vi "CS-4 Recall.vi"(8 "error in (no error)":errorcluster, 11 "VISA session":refnum<visa-resource-name>) -> (0 "error out":errorcluster, 1 "sweep rates":T2={"rate 0"=0.5, "rate 1"=0.25, "rate 2"=0.125, "rate 3"=10.0} {"rate 3" min=0.0 max=100.0 step=1.0 format="%.4f"; "rate 2" min=0.0 max=100.0 step=0.05 format="%.4f"; "rate 1" min=0.0 max=100.0 step=0.05 format="%.4f"; "rate 0" min=0.0 max=100.0 step=0.05 format="%.4f"}, 2 "range":cluster{"range 0":dbl, "range 1":dbl}={"range 0"=60.0, "range 1"=85.0} {"range 1" min=0.0 max=1000.0 format="%.3f"; "range 0" min=0.0 max=1000.0 step=1.0 format="%.3f"}, 3 "dup VISA session":refnum<visa-resource-name>, 4 "limits":T1={"Lower Current Limit"=-10.0, "Upper Current Limit"=10.0, "Voltage Limit"=5.0} {"Voltage Limit" min=0.0 max=5.0 format="%.2f"; "Upper Current Limit" min=-1000.0 max=1000.0 format="%.2f"; "Lower Current Limit" min=-1000.0 max=1000.0 format="%.1f"}, 5 "Units":enum16{"Amps", "Kilogauss", "Tesla"}(ring))   [LabVIEW 2016]
doc: "CS-4 Recall.vi uses the CS-4 driver VI's to recall setup information from a CS-4. This information includes display units, current sweep limits, and voltage limits. \n\nA VISA channel must be opened using CS-4 Initialize.vi before this VI is invoked."
panel:
  out "max supply current":dbl=100.0 format="%.3f"
  out "range 2 start":dbl format="%.3f"
  out "range 1 start":dbl format="%.3f"
  out "Cryo Logo copy":bool
  # "CRYOMAGNETICS, INC."
  # "Model CS-4"
  # "Magnet Power Supply Recall Settings"
  # "Sweep Ranges and Rates"
  # "Range 1"
  # "0.000"
  # "TO"
  # "Range 2"
  # "TO"
  # "Range 3"
  # "TO"
  # "Fast Mode"
  # "Limits"
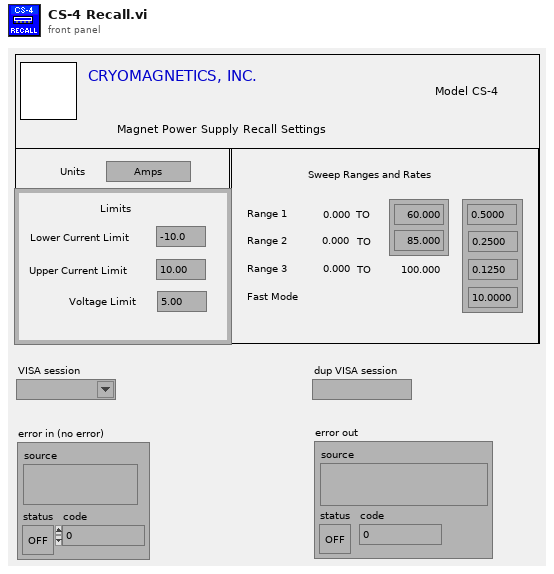
[diagram p1: front panel]
types:
  T1 = cluster{"Lower Current Limit":dbl, "Upper Current Limit":dbl, "Voltage Limit":dbl}
  T2 = cluster{"rate 0":dbl, "rate 1":dbl, "rate 2":dbl, "rate 3":dbl}
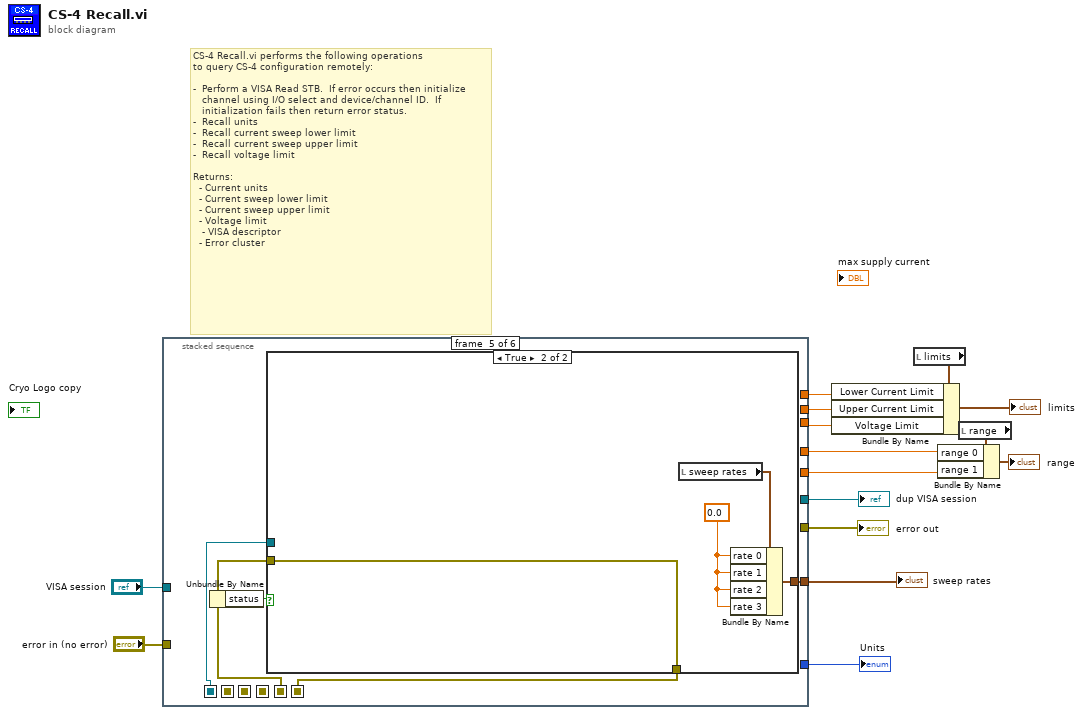
[diagram p0: block diagram]
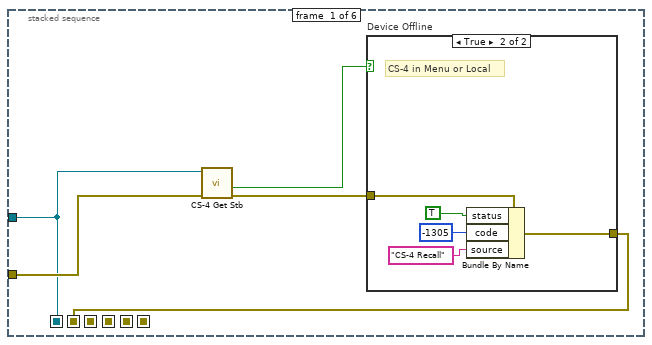
[diagram p2: hidden frame]
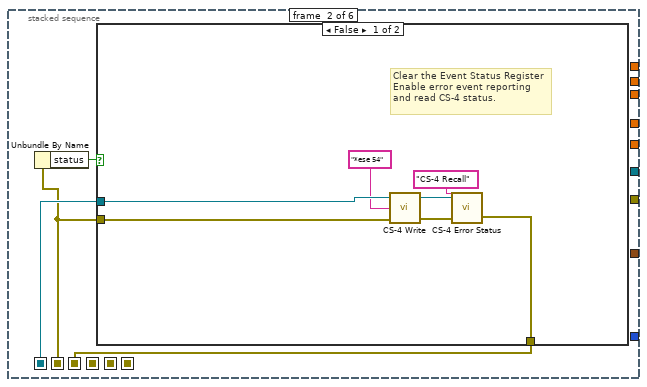
[diagram p4: hidden frame]
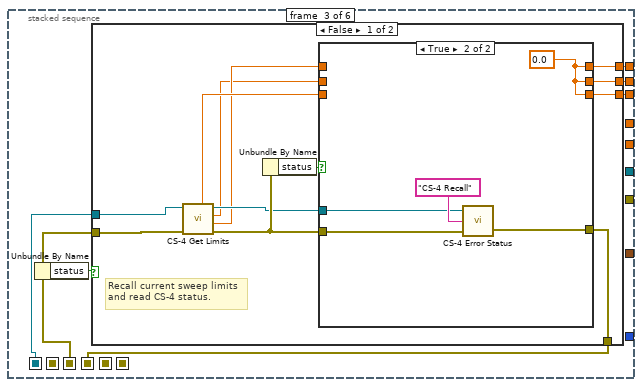
[diagram p6: hidden frame]
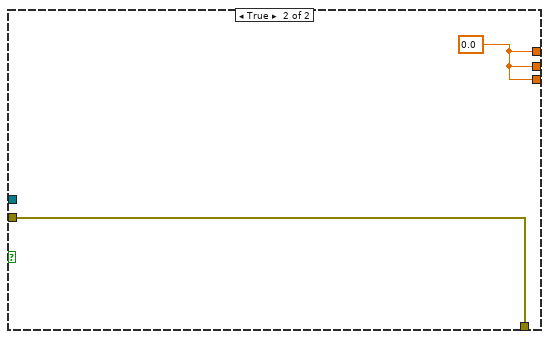
[diagram p8: hidden frame]
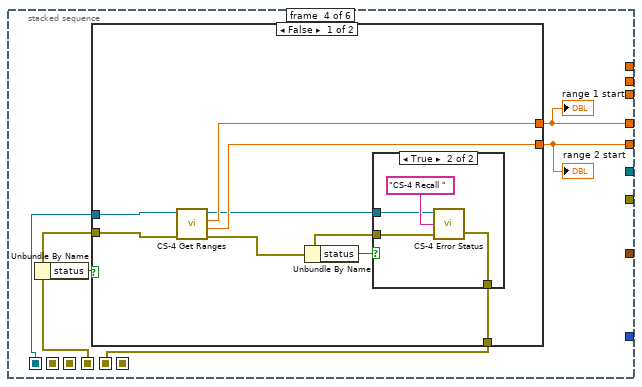
[diagram p9: hidden frame]
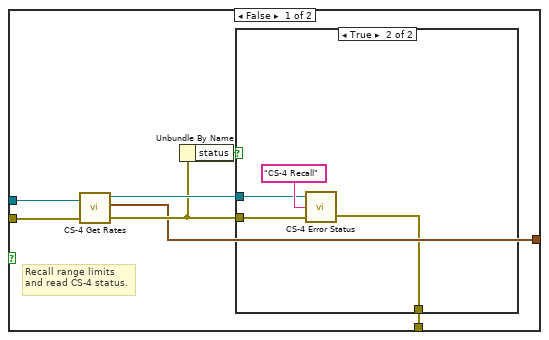
[diagram p12: hidden frame]
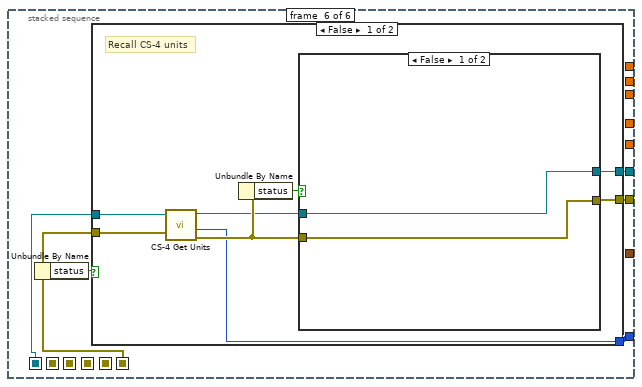
[diagram p14: hidden frame]
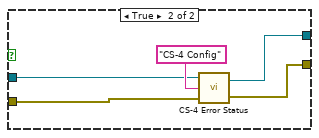
[diagram p15: hidden frame]
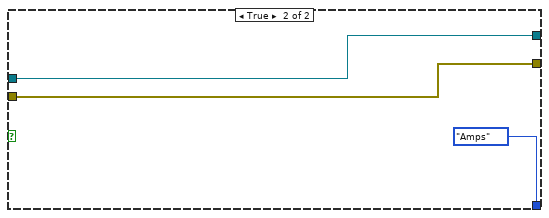
[diagram p16: hidden frame]
diagram:
  # "CS-4 Recall.vi performs the following operations\nto query CS-4 configuration remotely:\n\n-  Perform a VISA Read STB.  If error occurs then initialize \n   channel using I/O select and device/channel ID.  If \n   initialization fails then return error status.\n-  Recall units\n-  Recall current sweep lower limit\n-  Recall current sweep upper limit\n-  Recall voltage limit\n\nReturns:\n  - Current units\n  - Current sweep lower limit\n  - Current sweep upper limit\n  - Voltage limit\n   - VISA descriptor\n  - Error cluster"
  n1 = stacked-sequence {
    seq-local: [_ w27 _ _ _ _] -> [_ _ w41 _ _ _]
    seq-local: [w18 _ _ _ _ _] -> [_ w29 w44 w73 w93 w115]
    seq-local: [_ _ _ w69 _ _] -> [_ _ _ _ w92 _]
    seq-local: [w20 _ _ _ _ _] -> [_ w28 _ _ _ _]
    seq-local: [_ _ w40 _ _ _] -> [_ _ _ w70 _ _]
    seq-local: [_ _ _ _ w91 _] -> [_ _ _ _ _ w111]
    tunnel: "error in (no error)" -> [w19 _ _ _ _ _]
    tunnel: [_ _ _ _ _ w113] -> w14
    tunnel: [_ _ _ _ _ w112] -> w12
    tunnel: "VISA session" -> [w18 _ _ _ _ _]
    tunnel: [_ _ w43 _ _ _] -> w7
    tunnel: [_ _ w42 _ _ _] -> w10
    tunnel: [_ _ w39 _ _ _] -> w8
    tunnel: [_ _ _ _ _ w114] -> w11
    tunnel: [_ _ _ w72 _ _] -> w2
    tunnel: [_ _ _ w71 _ _] -> w3
    tunnel: [_ _ _ _ w90 _] -> w1
    frame #0 {
      n2 = call "CS-4 Get Stb.vi"("error in (no error)"=w19, "VISA session"=w18) -> ("error out"=w17:errorcluster, "Off Line"=w16:bool)  [unwired: 2 in, 2 out]
      n3 = case "Device Offline" shown="True" w16 {
        tunnel: [w21 w25] -> w20
        tunnel: w17 -> [w21 w26]
        frame False {
          # "CS-4 not in Menu or Local"
        }
        frame True {
          # "CS-4 in Menu or Local"
          n4 = Bundle By Name(cluster=w26, "status"=TRUE, "code"=-1305, "source"="CS-4 Recall") -> (w25:errorcluster)
        }
      }
    }
    frame #1 {
      n5 = Unbundle By Name(w28) -> ("status"=w30:bool)
      n6 = case shown="False" w30 {
        tunnel: w28 -> [w32 w38]
        tunnel: w29 -> [w33 _]
        tunnel: [w35 w38] -> w27
        frame False {
          # "Clear the Event Status Register\nEnable error event reporting\nand read CS-4 status."
          n7 = call "CS-4 Write.vi"("error in (no error)"=w32, "write buffer (\"\")"="*ese 54", "VISA session"=w33) -> ("error out"=w36:errorcluster, "dup VISA session"=w37:refnum<visa-resource-name>)  [unwired: 1 out]
          n8 = call "CS-4 Error Status.vi"("error in (no error)"=w36, "VI name"="CS-4 Recall", "VISA session"=w37) -> ("error out"=w35:errorcluster)  [unwired: 1 out]
        }
        frame True {
        }
      }
    }
    frame #2 {
      n9 = Unbundle By Name(w41) -> ("status"=w45:bool)
      n10 = case shown="False" w45 {
        tunnel: w41 -> [w53 w68]
        tunnel: w44 -> [w52 _]
        tunnel: [w57 w68] -> w40
        tunnel: [w55 w67] -> w43
        tunnel: [w54 w67] -> w42
        tunnel: [w48 w67] -> w39
        frame False {
          # "Recall current sweep limits\nand read CS-4 status."
          n11 = call "CS-4 Get Limits.vi"("error in (no error)"=w53, "VISA session"=w52) -> ("error out"=w51:errorcluster, "lower sweep limit"=w47:dbl, "upper sweep limit"=w46:dbl, "dup VISA session"=w50:refnum<visa-resource-name>, "voltage limit"=w49:dbl)  [unwired: 3 in]
          n12 = Unbundle By Name(w51) -> ("status"=w56:bool)
          n13 = case shown="True" w56 {
            tunnel: [w61 w66] -> w57
            tunnel: w51 -> [w61 w65]
            tunnel: w50 -> [_ w63]
            tunnel: [w59 w62] -> w55
            tunnel: [w58 w62] -> w54
            tunnel: w49 -> [w60 _]
            tunnel: [w60 w62] -> w48
            tunnel: w47 -> [w59 _]
            tunnel: w46 -> [w58 _]
            frame False {
            }
            frame True {
              w62 = 0.0
              n14 = call "CS-4 Error Status.vi"("error in (no error)"=w65, "VI name"="CS-4 Recall", "VISA session"=w63) -> ("error out"=w66:errorcluster)  [unwired: 1 out]
            }
          }
        }
        frame True {
          w67 = 0.0
        }
      }
    }
    frame #3 {
      n15 = Unbundle By Name(w70) -> ("status"=w74:bool)
      n16 = case shown="False" w74 {
        tunnel: w70 -> [w82 w89]
        tunnel: w73 -> [w76 _]
        tunnel: [w80 w89] -> w69
        tunnel: [w77 w88] -> w72
        tunnel: [w81 w88] -> w71
        frame False {
          n17 = call "CS-4 Get Ranges.vi"("error in"=w82, "VISA session"=w76) -> ("error out"=w79:errorcluster, "range 1"=w81:dbl, "range 0"=w77:dbl, "dup VISA session"=w75:refnum<visa-resource-name>)  [unwired: 2 in]
          n18 = Unbundle By Name(w79) -> ("status"=w78:bool)
          n19 = case shown="True" w78 {
            tunnel: w79 -> [w83 w86]
            tunnel: [w83 w85] -> w80
            tunnel: w75 -> [_ w84]
            frame False {
            }
            frame True {
              n20 = call "CS-4 Error Status.vi"("error in (no error)"=w86, "VI name"="CS-4 Recall ", "VISA session"=w84) -> ("error out"=w85:errorcluster)  [unwired: 1 out]
            }
          }
        }
        frame True {
          w88 = 0.0
        }
      }
      "range 1 start" <- w72
      "range 2 start" <- w71
    }
    frame #4 {
      n21 = Unbundle By Name(w92) -> ("status"=w94:bool)
      n22 = case shown="True" w94 {
        tunnel: w92 -> [w101 w110]
        tunnel: w93 -> [w100 _]
        tunnel: [w98 w110] -> w91
        tunnel: [w95 w107] -> w90
        frame False {
          # "Recall range limits\nand read CS-4 status."
          n23 = call "CS-4 Get Rates.vi"("error in (no error)"=w101, "VISA session"=w100) -> ("error out"=w96:errorcluster, "sweep rates"=w95:T2, "dup VISA session"=w97:refnum<visa-resource-name>)  [unwired: 5 in]
          n24 = Unbundle By Name(w96) -> ("status"=w99:bool)
          n25 = case shown="True" w99 {
            tunnel: w97 -> [_ w105]
            tunnel: w96 -> [w102 w104]
            tunnel: [w102 w103] -> w98
            frame False {
            }
            frame True {
              n26 = call "CS-4 Error Status.vi"("error in (no error)"=w104, "VI name"="CS-4 Recall", "VISA session"=w105) -> ("error out"=w103:errorcluster)  [unwired: 1 out]
            }
          }
        }
        frame True {
          w108 = 0.0
          n27 = local read "sweep rates"() -> (w109:T2)
          n28 = Bundle By Name(cluster=w109, "rate 0"=w108, "rate 1"=w108, "rate 2"=w108, "rate 3"=w108) -> (w107:T2)
        }
      }
    }
    frame #5 {
      n29 = Unbundle By Name(w111) -> ("status"=w116:bool)
      n30 = case shown="False" w116 {
        tunnel: w111 -> [w121 w134]
        tunnel: w115 -> [w122 w133]
        tunnel: [w124 w134] -> w113
        tunnel: [w117 enum16{"Amps", "Kilogauss", "Tesla"}."Amps" ("Units")] -> w114
        tunnel: [w118 w133] -> w112
        frame False {
          # "Recall CS-4 units"
          n31 = call "CS-4 Get Units.vi"("VISA session"=w122, "error in (no error)"=w121) -> ("dup VISA session"=w119:refnum<visa-resource-name>, "units"=w117:enum16{"Amps", "Kilogauss", "Tesla"}, "error out"=w120:errorcluster)  [unwired: 1 out]
          n32 = Unbundle By Name(w120) -> ("status"=w123:bool)
          n33 = case shown="False" w123 {
            tunnel: [w126 w130] -> w124
            tunnel: w120 -> [w126 w129]
            tunnel: w119 -> [w125 w128]
            tunnel: [w125 w127] -> w118
            frame False {
            }
            frame True {
              n34 = call "CS-4 Error Status.vi"("error in (no error)"=w129, "VI name"="CS-4 Config", "VISA session"=w128) -> ("error out"=w130:errorcluster, "dup VISA session"=w127:refnum<visa-resource-name>)
            }
          }
        }
        frame True {
        }
      }
    }
  }
  "error out" <- w14
  "sweep rates" <- w1
  "dup VISA session" <- w12
  "Units" <- w11
  n35 = local read "limits"() -> (w6:T1)
  n36 = Bundle By Name(cluster=w6, "Lower Current Limit"=w7, "Upper Current Limit"=w10, "Voltage Limit"=w8) -> (→"limits":T1)
  n37 = local read "range"() -> (w5:cluster{"range 0":dbl, "range 1":dbl})
  n38 = Bundle By Name(cluster=w5, "range 0"=w2, "range 1"=w3) -> (→"range":cluster{"range 0":dbl, "range 1":dbl})
